vi "sensor cmd config set.vi"(9 "value":u32, 10 "config_type":u32(ring) items=["CONFIG_ENABLE_ACCEL", "CONFIG_ENABLE_GYRO", "CONFIG_ENABLE_MAG", "CONFIG_ENABLE_WIRELESS", "CONFIG_ENABLE_SD", "CONFIG_WIRELESS_CHANNEL_0", "CONFIG_WIRELESS_CHANNEL_1", "CONFIG_WIRELESS_CHANNEL_2", "CONFIG_WIRELESS_CHANNEL_3", "CONFIG_WIRELESS_ADDR_ID", "CONFIG_WIRELESS_ADDR_BLOCK_0", "CONFIG_WIRELESS_ADDR_BLOCK_1", "CONFIG_WIRELESS_ADDR_BLOCK_2", "CONFIG_WIRELESS_ADDR_BLOCK_3", "CONFIG_WIRELESS_TIME_SLICE", "CONFIG_WIRELESS_PROTOCOL", "CONFIG_ACCEL_FULL_SCALE", "CONFIG_ALWAYS_OFF", "CONFIG_SPIN_MODE", "CONFIG_BATTERY_LED", "CONFIG_WIRELESS_LATENCY", "CONFIG_TEMP_SELECT", "CONFIG_OUTPUT_SELECT", "CONFIG_DECIMATION_SELECT", "CONFIG_BYPASS_DECIMATION", "CONFIG_EXTEND_LED", "CONFIG_MAG_SET_RESET", "CONFIG_LOCAL_TIMEZONE", "CONFIG_ENABLE_LED", "CONFIG_ENABLE_BUTTON", "CONFIG_BUTTON_MODE", "CONFIG_LABEL_0", "CONFIG_LABEL_1", "CONFIG_LABEL_2", "CONFIG_LABEL_3", "CONFIG_DEBUG_LED", "CONFIG_DEBUG_FILE", "CONFIG_BATTERY_CUTOFF"], 11 "device_handle":u32) -> (2 "function return":i32, 3 "device_handle out":u32)   [LabVIEW 2019, in "apdm.lvlib"]
doc: "APDM_EXPORT int apdm_sensor_cmd_config_set(apdm_device_handle_t device_handle, const enum APDMDeviceConfig config_type, const uint32_t value);"
uses:
  apdm.lvlib
  Lee Lab/CP FES Walking 2018/Code/Working/LabVIEW/apdm.dll
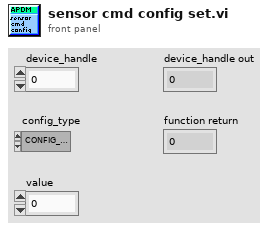
[diagram p1: front panel]
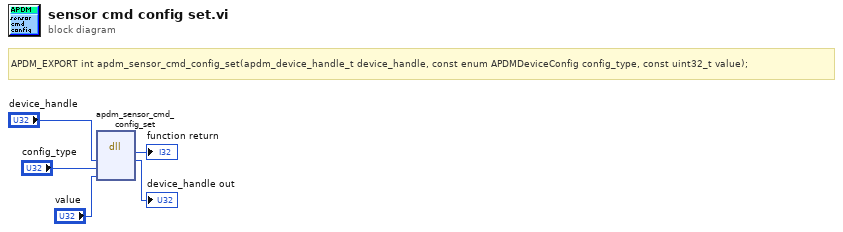
[diagram p0: block diagram]
diagram:
  # "APDM_EXPORT int apdm_sensor_cmd_config_set(apdm_device_handle_t device_handle, const enum APDMDeviceConfig config_type, const uint32_t value);"
  n1 = dll-call lib="C:/Users/jfalesi/Dropbox/Lee Lab/CP FES Walking 2018/Code/Working/LabVIEW/apdm.*" fn="apdm_sensor_cmd_config_set"("device_handle"="device_handle", "config_type"="config_type", "value"="value") -> (→"function return":i32, "device_handle"=→"device_handle out":u32)  [unwired: 5 in, 2 out]
